vi "UDMA_READ_FIFO.vi"(0 "TCP Network Connection in":refnum<k5>, 2 "N":u32=100, 5 "error in (no error)":errorcluster) -> (14 "TCP Network Connection out":refnum<k5>, 16 "Oscilloscope":u32[](graph), 18 "Status":u8[](array[numeric]), 19 "error out":errorcluster)   [LabVIEW 2019]
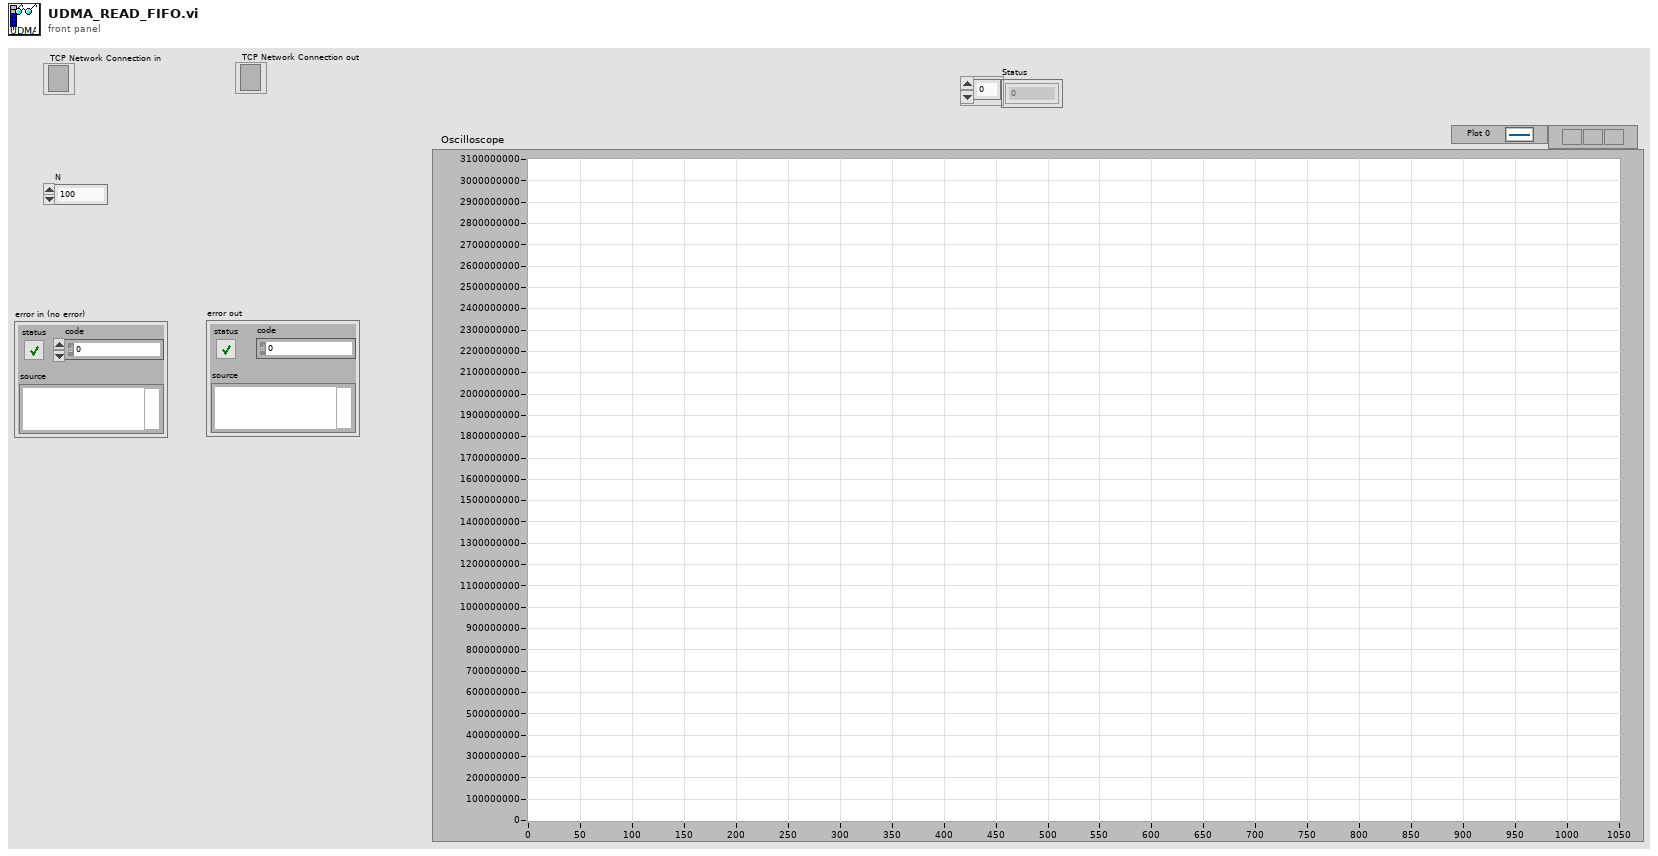
[diagram p1: front panel]
types:
  T1 = enum16{"big-endian, network order", "native, host order", "little-endian"}
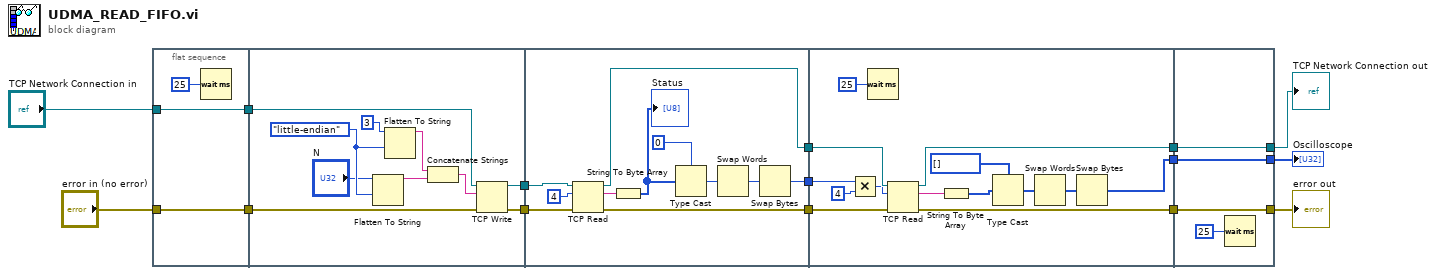
[diagram p0: block diagram]
diagram:
  n1 = flat-sequence {
    tunnel: [w17] -> w11
    tunnel: [w18] -> w10
    tunnel: "error in (no error)" -> [w18]
    tunnel: "TCP Network Connection in" -> [w17]
    tunnel: w11 -> [w28]
    tunnel: w10 -> [w27]
    tunnel: [w26] -> w5
    tunnel: [w25] -> w4
    tunnel: w5 -> [w36]
    tunnel: w4 -> [w39]
    tunnel: [w38] -> w3
    tunnel: [w29] -> w2
    tunnel: [w37] -> w1
    tunnel: w3 -> [w52]
    tunnel: w2 -> [w42]
    tunnel: [w51] -> w8
    tunnel: [w50] -> w7
    tunnel: [w40] -> w6
    tunnel: w1 -> [w53]
    tunnel: [w55] -> w9
    tunnel: [w56] -> w13
    tunnel: [w57] -> w12
    tunnel: w8 -> [w57]
    tunnel: w7 -> [w56]
    tunnel: w6 -> [w55]
    frame #0 {
      n2 = Wait (ms)(milliseconds to wait=u32 25) -> ()  [unwired: 1 out]
    }
    frame #1 {
      w23 = T1."little-endian" ("byte order (0:big-endian, network order)")
      n3 = Flatten To String(anything="N", byte order (0:big-endian, network order)=w23) -> (data string=w24:string)  [unwired: 2 in, 2 out]
      n4 = Flatten To String(anything=u32 3 ("element"), byte order (0:big-endian, network order)=w23) -> (data string=w21:string)  [unwired: 2 in, 2 out]
      n5 = Concatenate Strings(w21, w24) -> (w20:string)
      n6 = TCP Write(connection ID=w28, data in=w20, error in (no error)=w27) -> (connection ID out=w26:refnum<k5>, error out=w25:errorcluster)  [unwired: 1 in, 1 out]
    }
    frame #2 {
      n7 = TCP Read(connection ID=w36, bytes to read=4, error in (no error)=w39) -> (connection ID out=w37:refnum<k5>, data out=w35:string, error out=w38:errorcluster)  [unwired: 2 in]
      n8 = String To Byte Array(string=w35) -> (unsigned byte array=w33:u8[])
      "Status" <- w33
      n9 = Type Cast(type=u32 0 ("y"), x=w33) -> (*(type *) &x=w32:u32)
      n10 = Swap Words(1:w32) -> (0:w31:u32)
      n11 = Swap Bytes(anything=w31) -> (byte swapped=w29:u32)
    }
    frame #3 {
      n12 = Multiply(x=w42, y=u32 4) -> (x*y=w48:u32)
      n13 = Wait (ms)(milliseconds to wait=u32 25) -> ()  [unwired: 1 out]
      n14 = TCP Read(connection ID=w53, bytes to read=w48, error in (no error)=w52) -> (connection ID out=w51:refnum<k5>, data out=w41:string, error out=w50:errorcluster)  [unwired: 2 in]
      n15 = String To Byte Array(string=w41) -> (unsigned byte array=w46:u8[])
      n16 = Type Cast(type=u32[] [], x=w46) -> (*(type *) &x=w44:u32[])
      n17 = Swap Words(1:w44) -> (0:w43:u32[])
      n18 = Swap Bytes(anything=w43) -> (byte swapped=w40:u32[])
    }
    frame #4 {
      n19 = Wait (ms)(milliseconds to wait=u32 25) -> ()  [unwired: 1 out]
    }
  }
  "error out" <- w13
  "TCP Network Connection out" <- w12
  "Oscilloscope" <- w9
